vi "HandleVersionMutation_StaticCommunity.vi"(4 "To Version":u16, 6 "From Version":u16, 8 "error in (no error)":errorcluster, 10 "SerializableData in":variant, 11 "BlueSerializable in":refnum<class "BlueSerializable.lvclass">) -> (0 "error out":errorcluster, 2 "SerializableData out":variant, 3 "BlueSerializable out":refnum<class "BlueSerializable.lvclass">)   [LabVIEW 2020, in "BlueSerialization.lvlib" / "BlueSerializable.lvclass"]
uses:
  BlueSerializable.lvclass
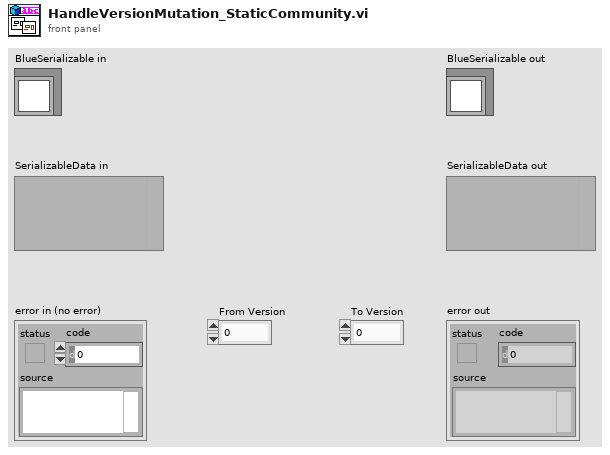
[diagram p1: front panel]
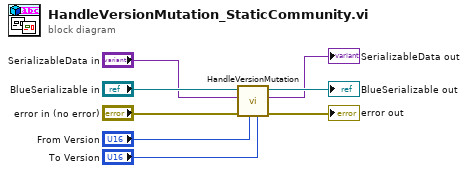
[diagram p0: block diagram]
diagram:
  n1 = call-dynamic "HandleVersionMutation.vi"("To Version"="To Version", "From Version"="From Version", "error in (no error)"="error in (no error)", "SerializableData in"="SerializableData in", "BlueSerializable in"="BlueSerializable in") -> ("error out"=→"error out":errorcluster, "SerializableData out"=→"SerializableData out":variant, "BlueSerializable out"=→"BlueSerializable out":refnum<class "BlueSerializable.lvclass">)  [unwired: 4 in]
